vi "waveform gen_DC_1.vi"(1 "Scale factor":u16=1, 2 "Boolean":bool, 3 "Exposure Time (s)":dbl(ring)=0.5 items=["0.2"=0.2, "0.5"=0.5, "1.0"=1.0, "4.0"=4.0, "8.0"=8.0], 4 "Laser Power%(0-100)":dbl=10.0) -> (0 "waveform":waveform(dbl)[](array[waveform]))   [LabVIEW 2018]
uses:
  <vilib>/Analysis/coordinate.llb/2D Cartesian Coordinate Rotation (Array).vi
  <vilib>/measure/NI_MABase.lvlib
  <vilib>/Analysis/NI_AALPro.lvlib
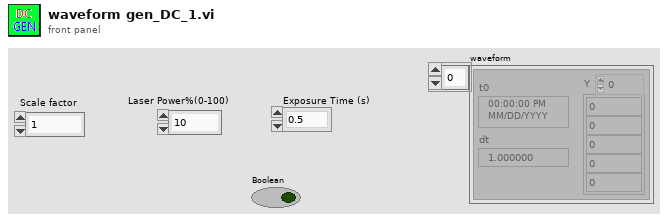
[diagram p1: front panel]
types:
  T1 = cluster{"Galvo/Pockels Cell Sampling Info":dbl, "#s":dbl}
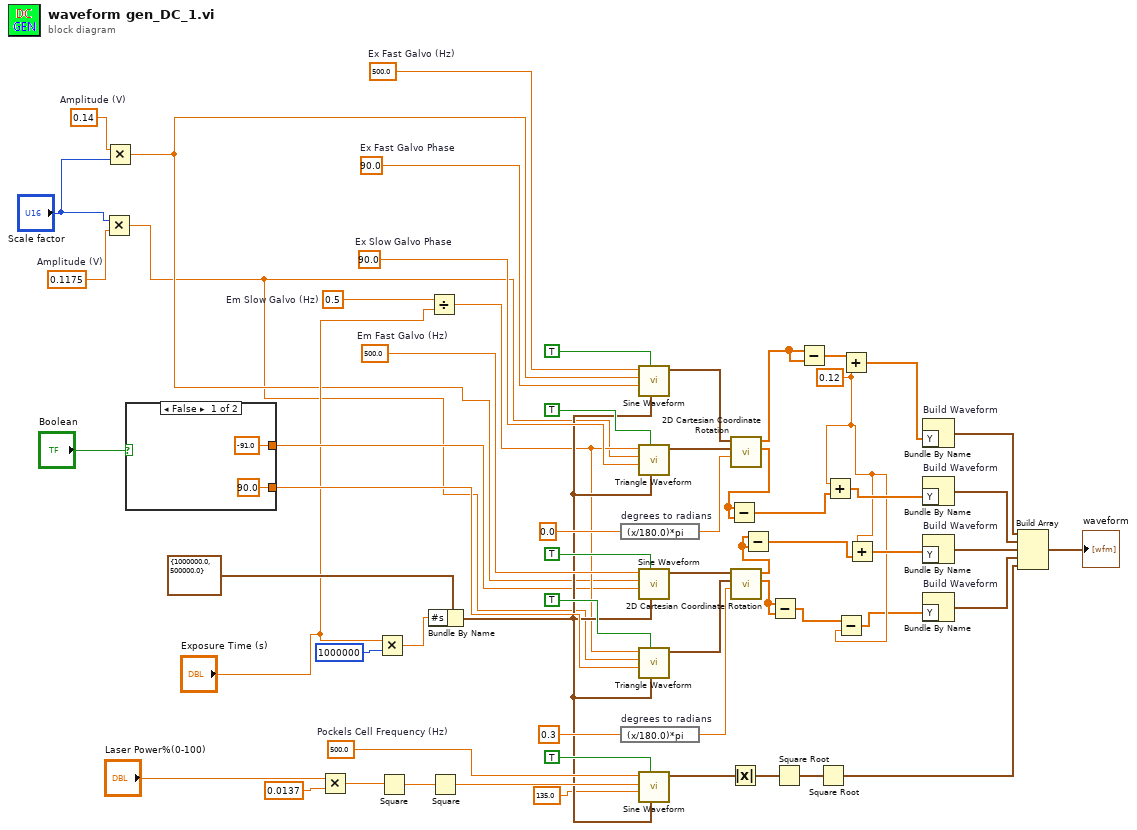
[diagram p0: block diagram]
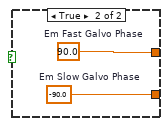
[diagram p2: hidden frame]
diagram:
  w2 = 0.12
  w26 = 0.5  # Em Slow Galvo (Hz)
  w15 = 0.1175  # Amplitude (V)
  w60 = 500.0  # Ex Fast Galvo (Hz)
  w18 = 0.14  # Amplitude (V)
  w59 = 500.0  # Pockels Cell Frequency (Hz)
  w57 = 500.0  # Em Fast Galvo (Hz)
  w53 = 90.0  # Ex Slow Galvo Phase
  w54 = 90.0  # Ex Fast Galvo Phase
  n1 = Multiply(x="Scale factor", y=w15) -> (x*y=w14:dbl)
  n2 = Multiply(x=w18, y="Scale factor") -> (x*y=w17:dbl)
  n3 = case shown="False" "Boolean" {
    tunnel: [90.0 ("Em Slow Galvo Phase") w65] -> w31
    tunnel: [-91.0 ("Em Fast Galvo Phase") w64] -> w23
    frame False {
    }
    frame True {
      w64 = 90.0  # Em Fast Galvo Phase
      w65 = -90.0  # Em Slow Galvo Phase
    }
  }
  n4 = Multiply(x="Laser Power%(0-100)", y=0.0137 ("data")) -> (x*y=w58:dbl)
  n5 = Multiply(x="Exposure Time (s)", y=1000000) -> (x*y=w27:dbl)
  n6 = Square(x=w58) -> (x^2=w46:dbl)
  n7 = Divide(x=w26, y="Exposure Time (s)") -> (x/y=w25:dbl)
  n8 = Bundle By Name(cluster=T1 {"Galvo/Pockels Cell Sampling Info"=1000000.0, "#s"=500000.0} ("Sampling Info"), "#s"=w27) -> (w29:T1)
  n9 = Square(x=w46) -> (x^2=w45:dbl)
  n10 = expression code="(x/180.0)*pi" "degrees to radians"(0.0 ("Ex Theta")) -> (w35:dbl)
  n11 = expression code="(x/180.0)*pi" "degrees to radians"(0.3 ("Em Theta")) -> (w32:dbl)
  n12 = call <vilib>:"Sine Waveform.vi"("sampling info"=w29, "reset signal"=TRUE, "phase"=w54, "amplitude"=w17, "frequency"=w60) -> ("signal out"=w43:waveform(dbl))  [unwired: 5 in, 1 out]
  n13 = call <vilib>:"Triangle Waveform.vi"("sampling info"=w29, "reset signal"=TRUE, "phase"=w53, "amplitude"=w14, "frequency"=w25) -> ("signal out"=w44:waveform(dbl))  [unwired: 5 in, 1 out]
  n14 = call <vilib>:"Sine Waveform.vi"("sampling info"=w29, "reset signal"=TRUE, "phase"=w23, "amplitude"=w17, "frequency"=w57) -> ("signal out"=w34:waveform(dbl))  [unwired: 5 in, 1 out]
  n15 = call <vilib>:"Triangle Waveform.vi"("sampling info"=w29, "reset signal"=TRUE, "phase"=w31, "amplitude"=w14, "frequency"=w25) -> ("signal out"=w39:waveform(dbl))  [unwired: 5 in, 1 out]
  n16 = call <vilib>:"Sine Waveform.vi"("sampling info"=w29, "reset signal"=TRUE, "phase"=135.0, "amplitude"=w45, "frequency"=w59) -> ("signal out"=w56:waveform(dbl))  [unwired: 5 in, 1 out]
  n17 = Absolute Value(x=w56) -> (abs(x)=w48:waveform(dbl))
  n18 = call-poly <vilib>:"2D Cartesian Coordinate Rotation.vi"("theta"=w35, "Y"=w44, "X"=w43) -> ("Y Out"=w12:dbl[], "X Out"=w13:dbl[])  [unwired: 6 in, 1 out]
  n19 = Subtract(x=w12, y=w12) -> (x-y=w8:dbl[])
  n20 = call-poly <vilib>:"2D Cartesian Coordinate Rotation.vi"("theta"=w32, "Y"=w39, "X"=w34) -> ("Y Out"=w4:dbl[], "X Out"=w11:dbl[])  [unwired: 6 in, 1 out]
  n21 = Subtract(x=w11, y=w11) -> (x-y=w6:dbl[])
  n22 = Subtract(x=w4, y=w4) -> (x-y=w3:dbl[])
  n23 = Square Root(x=w48) -> (sqrt(x)=w47:waveform(dbl))
  n24 = Subtract(x=w13, y=w13) -> (x-y=w10:dbl[])
  n25 = Square Root(x=w47) -> (sqrt(x)=w40:waveform(dbl))
  n26 = Add(x=w2, y=w8) -> (x+y=w7:dbl[])
  n27 = Subtract(x=w3, y=w2) -> (x-y=w1:dbl[])
  n28 = Add(x=w10, y=w2) -> (x+y=w9:dbl[])
  n29 = Add(x=w2, y=w6) -> (x+y=w5:dbl[])
  n30 = Bundle By Name "Build Waveform"("Y"=w9) -> (w42:waveform(dbl))  [unwired: 1 in]
  n31 = Bundle By Name "Build Waveform"("Y"=w7) -> (w41:waveform(dbl))  [unwired: 1 in]
  n32 = Bundle By Name "Build Waveform"("Y"=w5) -> (w37:waveform(dbl))  [unwired: 1 in]
  n33 = Bundle By Name "Build Waveform"("Y"=w1) -> (w38:waveform(dbl))  [unwired: 1 in]
  n34 = Build Array "Build Array"(w42, w41, w37, w38, w40) -> (→"waveform":waveform(dbl)[])
